vi "SelectMenu5.vi"(0 "XRef":T11, 1 "Tag":T7, 2 "Point":T10, 3 "Menu Type":T9, 4 "State In":T1) -> (14 "Reply":T6, 15 "Handled?":T8, 16 "Multi Object Popup Options":T5, 17 "Fatal Error Out":T4, 18 "State Out":T1)   [LabVIEW 2021, in "FirstXNode .xnode"]
uses:
  FirstXNode .xnode
  <vilib>/XNodeSupport/XNodeXNodeRef.ctl
  <vilib>/XNodeSupport/XNodeString.ctl
  <vilib>/XNodeSupport/XNodePoint.ctl
  <vilib>/XNodeSupport/XNodeInt.ctl
  <vilib>/XNodeSupport/XNodeMenuType.ctl
  State.ctl
  <vilib>/XNodeSupport/XNodeBounds.ctl
  <vilib>/XNodeSupport/XNodeStringArray.ctl
  <vilib>/XNodeSupport/XNodeBool.ctl
  <vilib>/XNodeSupport/XNodeMultiObjectPopupOptions.ctl
  <vilib>/XNodeSupport/XNodeErrorCluster.ctl
  <vilib>/XNodeSupport/NI_XNodeSupport.lvlib
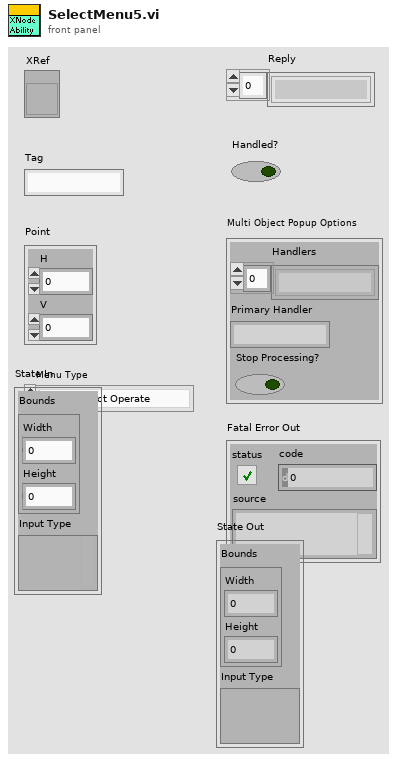
[diagram p1: front panel]
types:
  T1 = typedef "FirstXNode .xnode/State.ctl" = cluster{"Bounds":T2, "Input Type":variant}
  T2 = typedef "NI_XNodeSupport.lvlib/XNodeBounds.ctl" = cluster{"Width":T3, "Height":T3}
  T3 = typedef "NI_XNodeSupport.lvlib/XNodeInt.ctl" = i32
  T4 = typedef "NI_XNodeSupport.lvlib/XNodeErrorCluster.ctl" = errorcluster
  T5 = typedef "NI_XNodeSupport.lvlib/XNodeMultiObjectPopupOptions.ctl" = cluster{"Handlers":T6, "Primary Handler":T7, "Stop Processing?":T8}
  T6 = typedef "NI_XNodeSupport.lvlib/XNodeStringArray.ctl" = T7[]
  T7 = typedef "NI_XNodeSupport.lvlib/XNodeString.ctl" = string
  T8 = typedef "NI_XNodeSupport.lvlib/XNodeBool.ctl" = bool
  T9 = typedef "NI_XNodeSupport.lvlib/XNodeMenuType.ctl" = enum32{"Single Object Operate", "Single Object Popup", "Multi Object Popup Master", "Multi Object Popup Other"}
  T10 = typedef "NI_XNodeSupport.lvlib/XNodePoint.ctl" = cluster{"H":T3, "V":T3}
  T11 = typedef "NI_XNodeSupport.lvlib/XNodeXNodeRef.ctl" = refnum<vi>
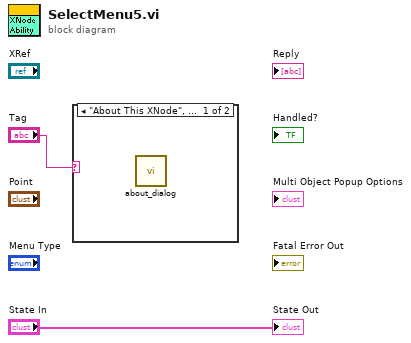
[diagram p0: block diagram]
diagram:
  n1 = case shown="\"About This XNode\", Default" "Tag" {
    frame "About This XNode", Default {
      n2 = call "about_dialog.vi"() -> ()  [unwired: 1 in]
    }
    frame "True" {
    }
  }
  "State Out" <- "State In"
